vi "ImageIvsPProcessPSTime.vi"(11 "Image in":refnum<class "Image.lvclass">) -> (1 "Added Image Intensity (I_new)":dbl[](array[numeric]), 2 "Array":T1(array[cluster]), 3 "Image out":refnum<class "Image.lvclass">)   [LabVIEW 2012, in "Image.lvclass"]
uses:
  classes/Image.lvclass
  classes/Image.lvclass/Image.ctl
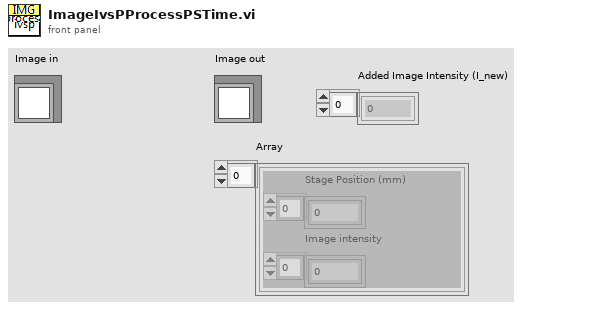
[diagram p1: front panel]
types:
  T1 = cluster{"Stage Position (mm)":dbl[], "Image intensity":dbl[]}[]
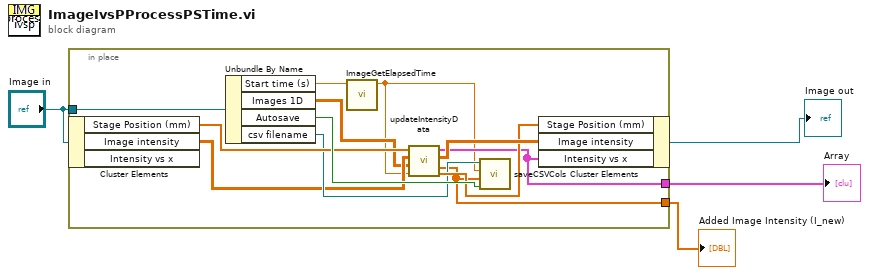
[diagram p0: block diagram]
diagram:
  n1 = in-place {
    in-place-border: "Image in" -> [w16]
    in-place-border: [w10] -> w2
    in-place-border: [w9] -> w1
    n2 = in-place-cluster #1("Image in") -> ("Stage Position (mm)"=w14:dbl[], "Image intensity"=w8:dbl[][])  [unwired: 1 out]
    n3 = Unbundle By Name(w16) -> ("Start time (s)"=w6:dbl, "Images 1D"=w7:dbl[][][], "Autosave"=w15:bool, "csv filename"=w11:path)
    n4 = call "ImageGetElapsedTime.vi"("start time"=w6) -> ("time elapsed (s)"=w5:dbl)  [unwired: 10 in]
    n5 = call "updateIntensityData.vi"("new x"=w5, "Images 2D"=w7, "Image Intensity (initial)"=w8, "x-axis (initial)"=w14) -> ("x-axis (final = initial + new)"=w12:dbl[], "Added Image Intensity (I_new)"=w10:dbl[], "Image Intensity (final = I_initial + I_new)"=w13:dbl[][], "Image Intensity vs x"=w9:cluster{dbl[], dbl[]}[])  [unwired: 4 in]
    n6 = call "saveCSVCols.vi"("Autosave"=w15, "y values"=w10, "x"=w5, "Image filename"=w11) -> ()  [unwired: 8 in]
    n7 = in-place-cluster #1("Stage Position (mm)"=w12, "Image intensity"=w13, "Intensity vs x"=w9) -> (→"Image out":refnum<class "Image.lvclass">)
  }
  "Array" <- w1
  "Added Image Intensity (I_new)" <- w2
